vi "Test_Calculate ORT.vi"(7 "Table Ref":refnum<vi>, 8 "ORT_MAX":dbl, 9 "Time Data":dbl[](array[numeric]), 10 "Current Data":dbl[](array[numeric]), 11 "Piezo Data":dbl[](array[numeric])) -> (2 "Pass?":bool, 3 "ORT [ms]":dbl)   [LabVIEW 2025]
panel:
  in  "error in (no error)":errorcluster
  out "error out":errorcluster
  out "T_0":dbl
  out "T_f":dbl
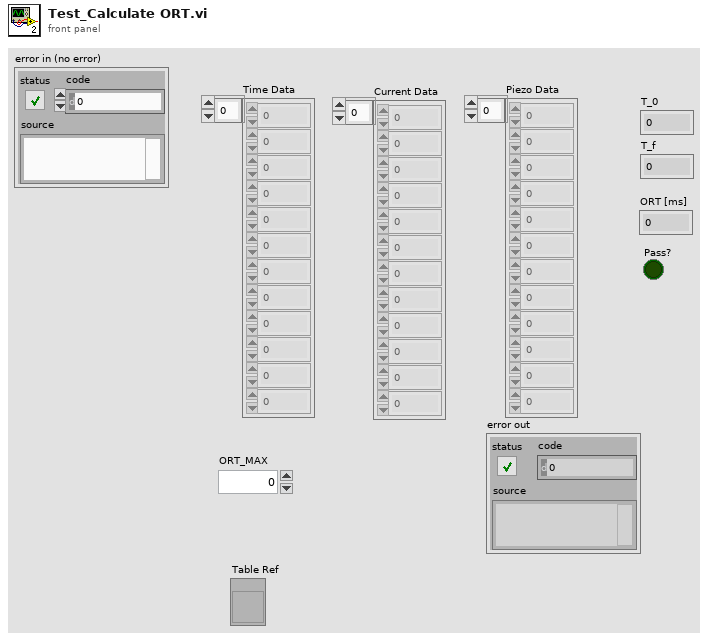
[diagram p1: front panel]
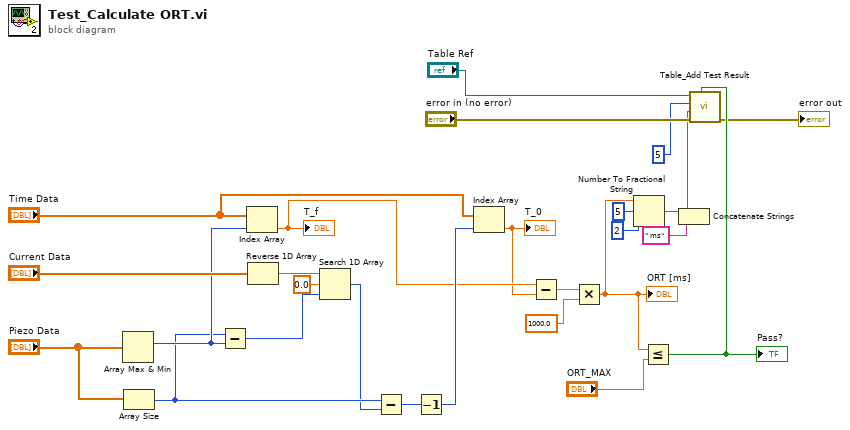
[diagram p0: block diagram]
diagram:
  n1 = Array Max & Min(array="Piezo Data") -> (max index (indices)=w25:i32)  [unwired: 3 out]
  n2 = Array Size(array="Piezo Data") -> (size(s)=w21:i32)
  n3 = Subtract(x=w21, y=w25) -> (x-y=w23:i32)
  n4 = Index Array(array="Time Data", index=w25) -> (element=w16:dbl)
  "T_f" <- w16
  n5 = Reverse 1D Array(array="Current Data") -> (reversed array=w24:dbl[])
  n6 = Search 1D Array(1D array=w24, element=0.0, start index (0)=w23) -> (index of element=w20:i32)
  n7 = Subtract(x=w21, y=w20) -> (x-y=w19:i32)
  n8 = Decrement(x=w19) -> (x-1=w17:i32)
  n9 = Index Array(array="Time Data", index=w17) -> (element=w15:dbl)
  "T_0" <- w15
  n10 = Subtract(x=w16, y=w15) -> (x-y=w14:dbl)
  n11 = Multiply(x=w14, y=1000.0) -> (x*y=w4:dbl)
  "ORT [ms]" <- w4
  n12 = Number To Fractional String(number=w4, width (-)=i16 5, precision (6)=i16 2) -> (F-format string=w3:string)  [unwired: 1 in]
  n13 = Less Or Equal?(x=w4, y="ORT_MAX") -> (x <= y?=w10:bool)
  "Pass?" <- w10
  n14 = Concatenate Strings(w3, " ms" ("string")) -> (w1:string)
  n15 = call "Table_Add Test Result.vi"("Boolean"=w10, "error in (no error)"="error in (no error)", "Test Result"=w1, "index (row)"=5, "Table in"="Table Ref") -> ("error out"=→"error out":errorcluster)  [unwired: 6 in]
